vi "MeasureIV.vi"(8 "Error In":errorcluster, 10 "Rf":dbl, 11 "LINX Resource":T1) -> (0 "Error Out":errorcluster, 1 "PD Current (A)":dbl, 2 "PD Voltage (V)":dbl, 3 "LINX Resource 2":T1)   [LabVIEW 2020]
uses:
  <vilib>/MakerHub/LINX/Private/Type Defs/LINX Ref.ctl
  <vilib>/MakerHub/LINX/Private/Type Defs/Platform.ctl
  <vilib>/MakerHub/LINX/Private/Type Defs/Interface.ctl
  <vilib>/MakerHub/LINX/Private/Device/Type Defs/LINX Device Config.ctl
  <vilib>/MakerHub/LINX/Private/Device/Type Defs/TCP Config.ctl
  <vilib>/MakerHub/LINX/Private/Device/Type Defs/Channels.ctl
  <vilib>/MakerHub/LINX/Public/Peripherals/Analog/Analog Read 1 Chan.vi
  <vilib>/MakerHub/LINX/Public/Peripherals/Analog/Analog Read N Chans.vi
  <vilib>/MakerHub/LINX/Private/Local IO/LinxAnalogRead.vi
  <vilib>/MakerHub/LINX/Public/Utilities/Check Channel.vi
  <vilib>/MakerHub/LINX/Private/Utilties/Generate Error.vi
  <vilib>/MakerHub/LINX/LMH-LINX.lvlib
  <vilib>/MakerHub/LINX/Private/Device/Device.lvlib
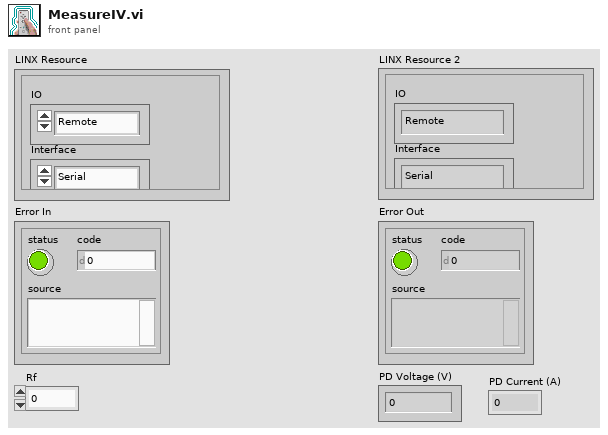
[diagram p1: front panel]
types:
  T1 = typedef "LMH-LINX.lvlib/LINX Ref.ctl" = cluster{"IO":T2, "Interface":T3, "LINX Device Config":T4}
  T2 = typedef "LMH-LINX.lvlib/Platform.ctl" = enum16{"Remote", "Local"}
  T3 = typedef "LMH-LINX.lvlib/Interface.ctl" = enum16{"Serial", "TCP"}
  T4 = typedef "LMH-LINX.lvlib/Device.lvlib/LINX Device Config.ctl" = cluster{"Interface":T3, "COM Port":refnum<visa-resource-name>, "TCP Configuration":T5, "Device Family":u8, "Device ID":u8, "Device Name":string, "TCP Ref":refnum<k5>, "Channels":T6}
  T5 = typedef "LMH-LINX.lvlib/Device.lvlib/TCP Config.ctl" = cluster{"IP Address":string, "Port":u16}
  T6 = typedef "LMH-LINX.lvlib/Channels.ctl" = cluster{"DI":u8[], "DO":u8[], "AI":u8[], "AO":u8[], "PWM":u8[], "QE":u8[], "UART":u8[], "I2C 2":u8[], "SPI":u8[], "CAN":u8[], "Servo":u8[], "AI Ref (V)":dbl, "AI Resolution (Bits)":u8, "AO Ref (V)":dbl, "AO Resolution (Bits)":u8}
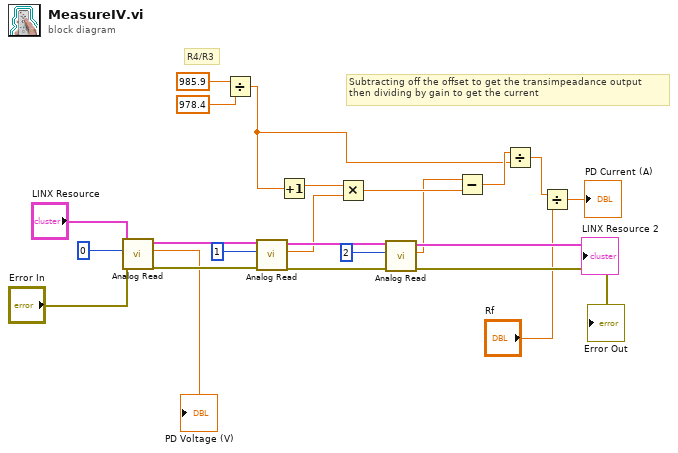
[diagram p0: block diagram]
diagram:
  # "Subtracting off the offset to get the transimpeadance output\nthen dividing by gain to get the current"
  # "R4/R3"
  n1 = call-poly <vilib>:"Analog Read.vi"("Error In"="Error In", "Analog Channel"=u8 0, "LINX Resource"="LINX Resource") -> ("Error Out"=w20:errorcluster, "Voltage"=→"PD Voltage (V)":dbl, "LINX Resource"=w23:T1)  [unwired: 5 in, 1 out]
  n2 = Divide(x=985.9, y=978.4) -> (x/y=w1:dbl)
  n3 = call-poly <vilib>:"Analog Read.vi"("Error In"=w20, "Analog Channel"=u8 1, "LINX Resource"=w23) -> ("Error Out"=w21:errorcluster, "Voltage"=w8:dbl, "LINX Resource"=w22:T1)  [unwired: 5 in, 1 out]
  n4 = Increment(x=w1) -> (x+1=w9:dbl)
  n5 = Multiply(x=w9, y=w8) -> (x*y=w7:dbl)
  n6 = call-poly <vilib>:"Analog Read.vi"("Error In"=w21, "Analog Channel"=u8 2, "LINX Resource"=w22) -> ("Error Out"=→"Error Out":errorcluster, "Voltage"=w4:dbl, "LINX Resource"=→"LINX Resource 2":T1)  [unwired: 5 in, 1 out]
  n7 = Subtract(x=w4, y=w7) -> (x-y=w3:dbl)
  n8 = Divide(x=w3, y=w1) -> (x/y=w2:dbl)
  n9 = Divide(x=w2, y="Rf") -> (x/y=→"PD Current (A)":dbl)
